vi "Exercise3-5.vi"() -> ()   [LabVIEW 2014]
panel:
  out "Warning Text":string
  out "Warning?":bool
  in  "Current Temp":dbl
  in  "Max Temp":dbl
  in  "Min Temp":dbl
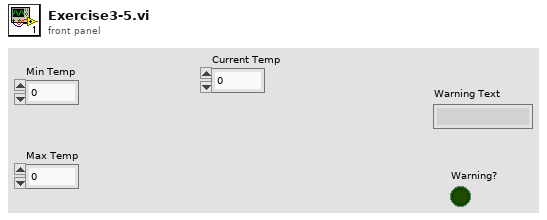
[diagram p1: front panel]
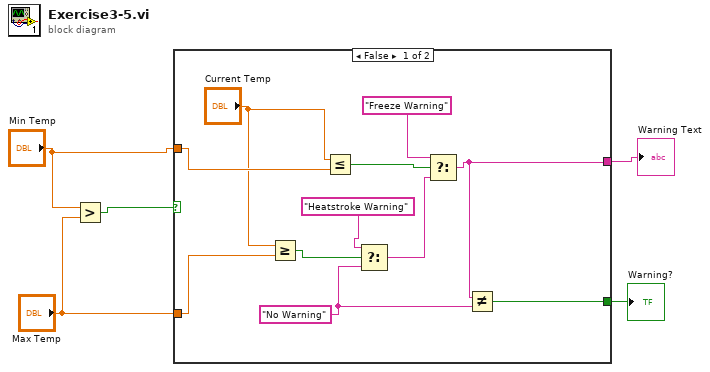
[diagram p0: block diagram]
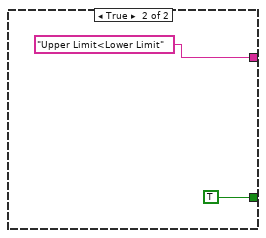
[diagram p2: hidden frame]
diagram:
  n1 = Greater?(x="Min Temp", y="Max Temp") -> (0:w5:bool)
  n2 = case shown="False" w5 {
    tunnel: "Max Temp" -> [w14 _]
    tunnel: "Min Temp" -> [w13 _]
    tunnel: [w7 "Upper Limit<Lower Limit"] -> w1
    tunnel: [w6 TRUE] -> w2
    frame False {
      w8 = "No Warning"
      n3 = Greater Or Equal?(x="Current Temp", y=w14) -> (x >= y?=w15:bool)
      n4 = Less Or Equal?(x="Current Temp", y=w13) -> (x <= y?=w16:bool)
      n5 = Select(t="Heatstroke Warning", s=w15, f=w8) -> (s? t:f=w11:string)
      n6 = Select(t="Freeze Warning", s=w16, f=w11) -> (s? t:f=w7:string)
      n7 = Not Equal?(x=w7, y=w8) -> (x != y?=w6:bool)
    }
    frame True {
    }
  }
  "Warning?" <- w2
  "Warning Text" <- w1
